vi "Stream to Image Files (Optimized Performance) ajg.vi"() -> ()   [LabVIEW 2020]
doc: "The Stream to Image Files (Optimized Performance) example shows how to save images to PNG files in parallel when using a ring acquisition. Images acquired from a camera are stored in a ring buffer and references to each image are pushed to a queue. Each worker loop removes a reference from the queue and saves the image to disk. When processing is complete, <B>IMAQdx Release Image</B> must be called in order to free space in the ring buffer."
uses:
  <vilib>/vision/driver/IMAQdx.llb/IMAQdx Acquisition Mode.ctl
  <vilib>/vision/Image Controls.llb/IMAQ Image.ctl
  <vilib>/vision/driver/IMAQdx.llb/IMAQdx Buffer Number Mode.ctl
  <vilib>/Utility/High Resolution Relative Seconds.vi
  <vilib>/vision/driver/NI_Vision_Acquisition_Software.lvlib
  <resource>/objmgr/imaqdx.rc
panel:
  in  "Tab Control":enum32{"Main", "Instructions"}(tab)
  in  "Stop":bool
  in  "Camera Name":refnum<k21> caption="IMAQdx Session"
  in  "Number of Images":i32=30
  out "Images Behind":i32
  out "Write Speed":dbl(graph) caption="Image File Write Speed"
  in  "Number of Workers":u8=3 min=1 max=3
  out "Images Acquired Per Second":dbl
  out "Images Saved Per Second":dbl
  in  "Skip Count":u32
  in  "Destination Folder":path
  in  "ms between datasets":dbl
  out "error out 2":errorcluster
  in  "Stopped":bool
  # "Overview: Stream images to disk in parallel. Creates folders within destinatio folder and puts 10,000 files in each folder.\nRequirements: Vision Acquisition Software\nInstructions:\n1. Select the Camera Name\n2. Run the VI\n3. Reduce the Number of Workers to see if the streaming of images can keep up with fewer workers.\n4. Increase the Skip Count if Images Behind is greater than 0.\n5. Use the skip count to skip acquiring some images so the image logging can avoid getting behind.\n6. max workers is 3"
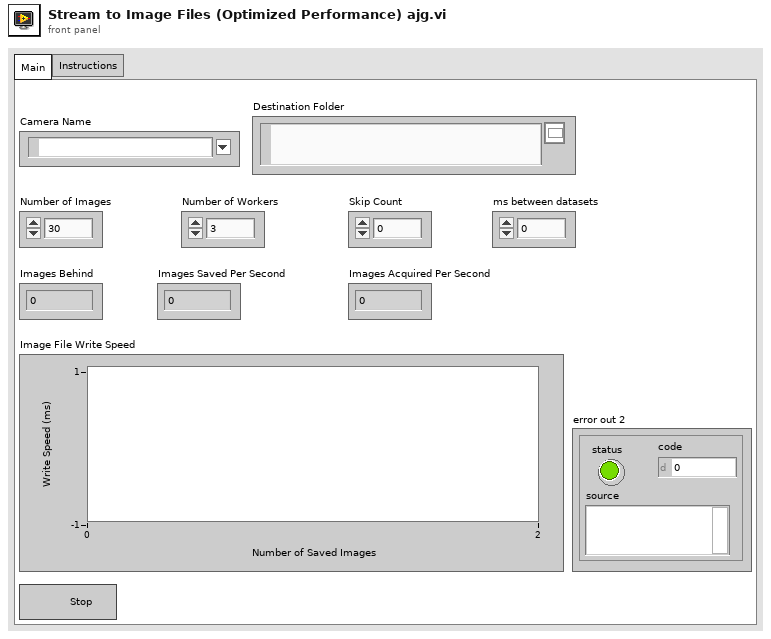
[diagram p1: front panel]
types:
  T1 = typedef "IMAQ Image.ctl" = refnum<image>
  T2 = typedef "NI_Vision_Acquisition_Software.lvlib/IMAQdx Acquisition Mode.ctl" = enum32{"One Shot", "Continuous"}
  T3 = typedef "NI_Vision_Acquisition_Software.lvlib/IMAQdx Buffer Number Mode.ctl" = enum32{"Next", "Last", "Buffer Number", "Every", "Last New"}
  T4 = typedef "IMAQdx.ctl" = refnum<k21>
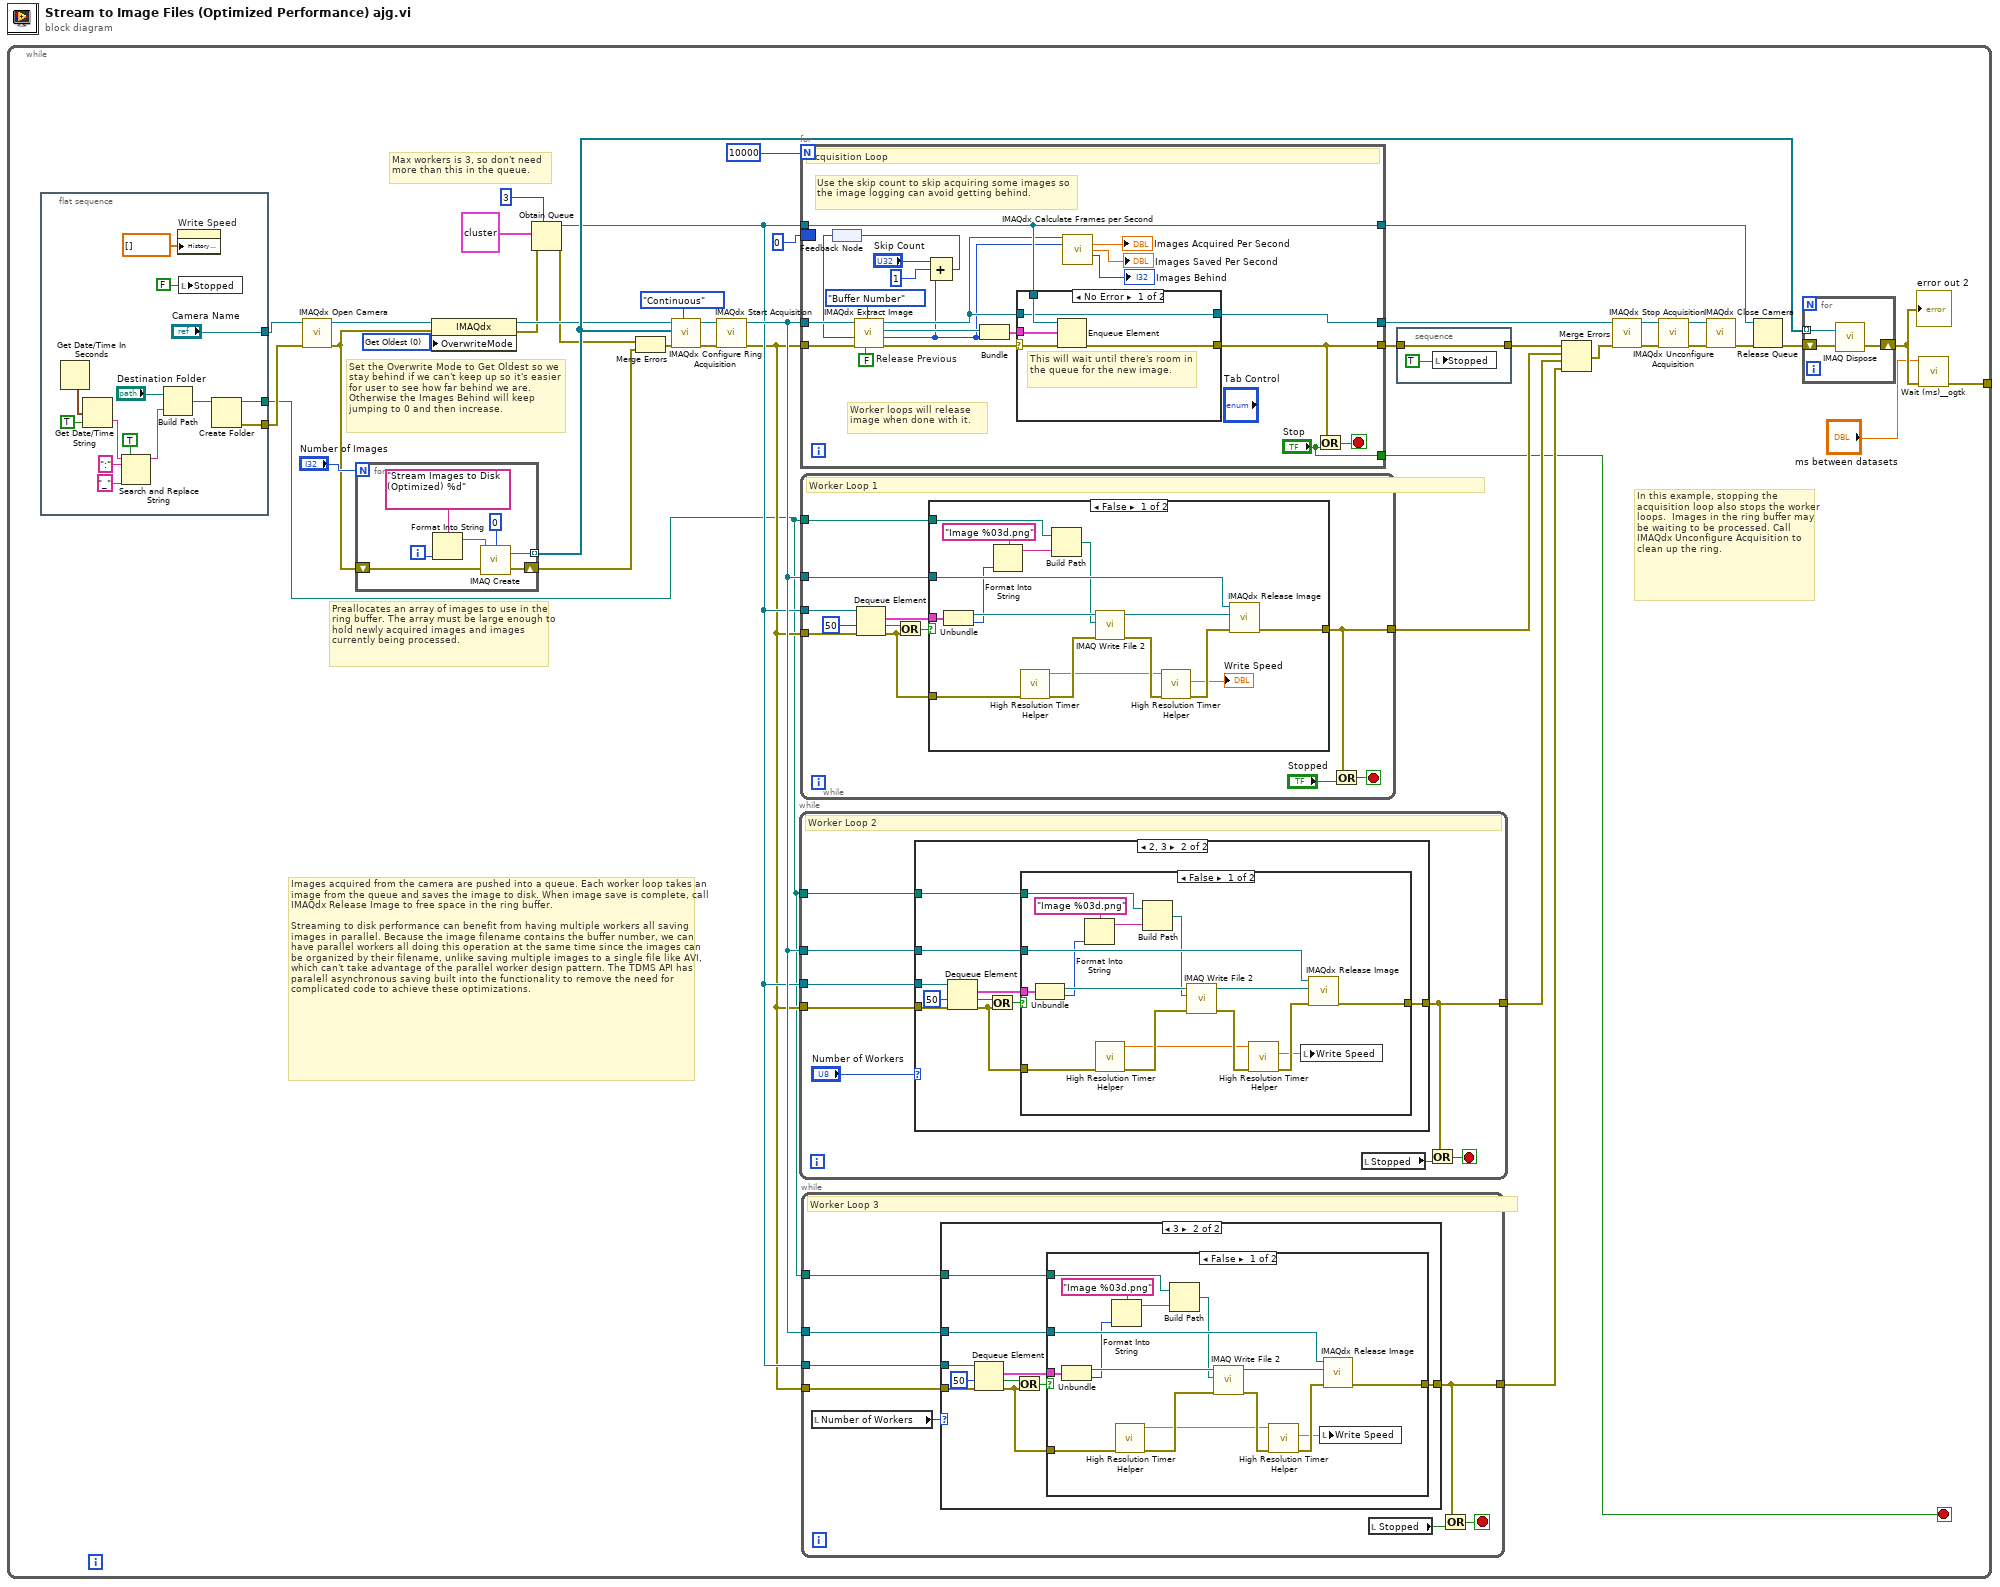
[diagram p0: block diagram]
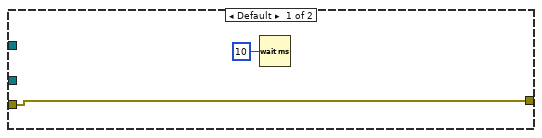
[diagram p3: hidden frame]
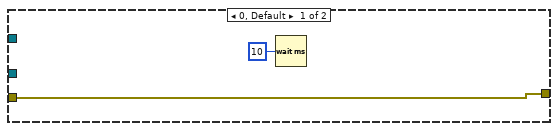
[diagram p5: hidden frame]
diagram:
  n1 = while {
    tunnel: [w3] -> _
    stop <- w10 stop-if-true
    w16 = u32 0 items=["Get Oldest"=0, "Fail"=2, "Get Newest"=3] ("OverwriteMode")
    # "Set the Overwrite Mode to Get Oldest so we stay behind if we can't keep up so it's easier for user to see how far behind we are. Otherwise the Images Behind will keep jumping to 0 and then increase."
    # "Max workers is 3, so don't need more than this in the queue."
    # "In this example, stopping the acquisition loop also stops the worker loops.  Images in the ring buffer may be waiting to be processed. Call IMAQdx Unconfigure Acquisition to clean up the ring."
    # "Images acquired from the camera are pushed into a queue. Each worker loop takes an image from the queue and saves the image to disk. When image save is complete, call IMAQdx Release Image to free space in the ring buffer. \n\nStreaming to disk performance can benefit from having multiple workers all saving images in parallel. Because the image filename contains the buffer number, we can have parallel workers all doing this operation at the same time since the images can be organized by their filename, unlike saving multiple images to a single file like AVI, which can't take advantage of the parallel worker design pattern. The TDMS API has paralell asynchronous saving built into the functionality to remove the need for complicated code to achieve these optimizations."
    # "Preallocates an array of images to use in the ring buffer. The array must be large enough to hold newly acquired images and images currently being processed."
    n2 = flat-sequence {
      tunnel: ["Camera Name"] -> w6
      tunnel: [w42] -> w5
      tunnel: [w41] -> w4
      frame #0 {
        n3 = Get Date/Time In Seconds() -> (seconds since 1Jan1904=w47:timestamp)
        n4 = Get Date/Time String(seconds (now)=w47, want seconds? (F)=TRUE) -> (time string=w48:string)  [unwired: 1 in, 1 out]
        n5 = Search and Replace String(replace all?=TRUE ("replace all? (F)"), input string=w48, search string=":", replace string="_" ("replace string (\"\")")) -> (result string=w51:string)  [unwired: 4 in, 3 out]
        n6 = Build Path(base path="Destination Folder", name or relative path=w51) -> (appended path=w50:path)
        n7 = property on="Write Speed" class="WFChart (strict)"("History Data"=dbl[] []) -> ()  [unwired: 2 in, 2 out]
        n8 = local write "Stopped"(FALSE ("Stop")) -> ()
        n9 = Create Folder(path (use dialog)=w50) -> (created path=w41:path, error out=w42:errorcluster)  [unwired: 2 in, 1 out]
      }
    }
    n10 = call <vilib>:"IMAQdx Open Camera.vi"("error in"=w5, "Session In"=w6) -> ("error out"=w15:errorcluster, "Session Out"=w17:T4)  [unwired: 1 in, 7 out]
    n11 = for {
      N: "Number of Images" -> [_]
      tunnel: [w196] -> w30 mode=indexing
      shift-right: [w195] -> w12
      shift-left: w15 -> [w197]
      i -> [w194]
      n12 = Format Into String(format string="Stream Images to Disk (Optimized) %d" ("Image Name"), w194) -> (resulting string=w193:string)  [unwired: 2 in, 1 out]
      n13 = call "IMAQ Create"("Border Size"=0, "Image Name"=w193, "error in (no error)"=w197) -> ("New Image"=w196:T1, "error out"=w195:errorcluster)  [unwired: 1 in, 1 out]
    }
    n14 = property class="IMAQdx"(reference=w17, error in=w15, "OverwriteMode"=w16) -> (error out=w14:errorcluster)  [unwired: 1 out]
    n15 = Obtain Queue(max queue size (-1, unlimited)=3, element data type=cluster{"Image Out":T1, "Buffer Number Out":u32} {"Image Out"=refnum, "Buffer Number Out"=0}, error in (no error)=w14) -> (queue out=w21:refnum<queue>, error out=w13:errorcluster)  [unwired: 2 in, 1 out]
    n16 = Merge Errors(w13, w12) -> (w33:errorcluster)
    n17 = call <vilib>:"IMAQdx Configure Ring Acquisition.vi"("Mode"=IMAQdx_Acquisition_Mode."Continuous" ("Continuous?"), "error in"=w33, "Images"=w30, "Session In"=w17) -> ("error out"=w9:errorcluster, "Session Out"=w36:T4)  [unwired: 5 in, 1 out]
    n18 = call <vilib>:"IMAQdx Start Acquisition.vi"("error in"=w9, "Session In"=w36) -> ("error out"=w20:errorcluster, "Session Out"=w22:T4)  [unwired: 8 out]
    n19 = while {
      tunnel: w21 -> [w124]
      tunnel: w22 -> [w126]
      tunnel: w20 -> [w123]
      tunnel: w4 -> [w125]
      tunnel: [w122] -> w23
      stop <- w127 stop-if-true
      # "Worker Loop 2"
      n20 = case shown="2, 3" "Number of Workers" {
        tunnel: w126 -> [_ w134]
        tunnel: w125 -> [_ w133]
        tunnel: w124 -> [_ w132]
        tunnel: w123 -> [w129 w131]
        tunnel: [w129 w130] -> w122
        frame 0, Default {
          n21 = Wait (ms)(milliseconds to wait=u32 10) -> ()  [unwired: 1 out]
        }
        frame 2, 3 {
          n22 = Dequeue Element(queue=w132, timeout in ms (-1)=50 ("timeout in ms"), error in (no error)=w131) -> (element=w136:cluster{"Image Out":T1, "Buffer Number Out":u32}, timed out?=w138:bool, error out=w139:errorcluster)  [unwired: 1 out]
          n23 = Or(x=w138, y=w139) -> (x .or. y?=w137:bool)
          n24 = case shown="False" w137 {
            tunnel: w139 -> [w145 w156]
            tunnel: w136 -> [w155 _]
            tunnel: [w154 w156] -> w130
            tunnel: w134 -> [w153 _]
            tunnel: w133 -> [w150 _]
            frame False {
              n25 = Unbundle(w155) -> ("Image Out"=w152:T1, "Buffer Number Out"=w147:u32)
              n26 = Format Into String(format string="Image %03d.png", w147) -> (resulting string=w149:string)  [unwired: 2 in, 1 out]
              n27 = call "High Resolution Timer Helper.vi"("error in (no error)"=w145) -> ("error out"=w144:errorcluster, "Current Time"=w141:dbl)  [unwired: 8 in, 1 out]
              n28 = Build Path(base path=w150, name or relative path=w149) -> (appended path=w146:path)
              n29 = call-poly "IMAQ Write File 2"("error in (no error)"=w144, "File Path"=w146, "Image"=w152) -> ("error out"=w143:errorcluster, "Image Out (duplicate)"=w151:T1)  [unwired: 7 in]
              n30 = call "High Resolution Timer Helper.vi"("error in (no error)"=w143, "Previous Time"=w141) -> ("error out"=w142:errorcluster, "Time Difference (ms)"=w140:dbl)  [unwired: 7 in, 1 out]
              n31 = local write "Write Speed"(w140) -> ()
              n32 = call <vilib>:"IMAQdx Release Image.vi"("error in"=w142, "Image"=w151, "Session In"=w153) -> ("error out"=w154:errorcluster)  [unwired: 7 in, 1 out]
            }
            frame True {
              # "Empty queue or error.\nNothing to process."
            }
          }
        }
      }
      n33 = local read "Stopped"() -> (w120:bool)
      n34 = Or(x=w122, y=w120) -> (x .or. y?=w127:bool)
    }
    n35 = for {
      N: 10000 ("Max Files") -> [_]
      tunnel: w20 -> [w75]
      tunnel: w22 -> [w72]
      tunnel: w21 -> [w68]
      tunnel: [w67] -> w29
      tunnel: [w66] -> w26
      tunnel: [w68] -> w31
      tunnel: ["Stop"] -> w10
      border: u32 0 -> [_]
      stop <- w56 stop-if-true
      w73 = FALSE  # Release Previous
      # "Use the skip count to skip acquiring some images so the image logging can avoid getting behind."
      # "Worker loops will release image when done with it."
      # "Acquisition Loop"
      n36 = feedback #1() -> (w64:u32)
      n37 = call <vilib>:"IMAQdx Extract Image.vi"("Release Previous (true)"=w73, "Buffer Number Mode (Next)"=IMAQdx_Buffer_Number_Mode."Buffer Number" ("Buffer Number Mode"), "error in"=w75, "Buffer Number In"=w64, "Session In"=w72) -> ("error out"=w71:errorcluster, "Buffer Number Out"=w57:u32, "Image Out"=w70:T1, "Session Out"=w58:T4)  [unwired: 3 in]
      n38 = Compound Arithmetic op=ADD("Skip Count", u32 1 ("value"), w57) -> (w65:u32)
      n39 = feedback-in #1(w65) -> ()
      n40 = Bundle("Image Out"=w70, "Buffer Number Out"=w57) -> (w69:cluster{"Image Out":T1, "Buffer Number Out":u32})  [unwired: 1 in]
      n41 = case shown="No Error" w71 {
        selector: w71 -> [w80 w81]
        tunnel: [w76 w82] -> w67
        tunnel: w58 -> [w76 w82]
        tunnel: w69 -> [w79 _]
        tunnel: w68 -> [w78 _]
        tunnel: [w77 w81] -> w66
        frame No Error {
          # "This will wait until there's room in the queue for the new image."
          n42 = Enqueue Element(queue=w78, element=w79, error in (no error)=w80) -> (error out=w77:errorcluster)  [unwired: 1 in, 2 out]
        }
        frame Error {
        }
      }
      n43 = call <vilib>:"IMAQdx Calculate Frames per Second.vi"("Session In"=w58, "Buffer Number"=w57) -> ("Acquired Frames per Second"=→"Images Acquired Per Second":dbl, "Processed Frames per Second"=→"Images Saved Per Second":dbl, "Images Behind"=→"Images Behind":i32)  [unwired: 7 in, 4 out]
      n44 = Or(x=w66, y="Stop") -> (x .or. y?=w56:bool)
    }
    n45 = while {
      tunnel: w21 -> [w165]
      tunnel: w22 -> [w167]
      tunnel: w20 -> [w164]
      tunnel: w4 -> [w166]
      tunnel: [w163] -> w24
      stop <- w173 stop-if-true
      # "Worker Loop 1"
      n46 = Dequeue Element(queue=w165, timeout in ms (-1)=50 ("timeout in ms"), error in (no error)=w164) -> (element=w169:cluster{"Image Out":T1, "Buffer Number Out":u32}, timed out?=w171:bool, error out=w172:errorcluster)  [unwired: 1 out]
      n47 = Or(x=w171, y=w172) -> (x .or. y?=w170:bool)
      n48 = case shown="False" w170 {
        tunnel: w172 -> [w179 w190]
        tunnel: w169 -> [w189 _]
        tunnel: [w188 w190] -> w163
        tunnel: w167 -> [w187 _]
        tunnel: w166 -> [w184 _]
        frame False {
          n49 = Unbundle(w189) -> ("Image Out"=w186:T1, "Buffer Number Out"=w181:u32)
          n50 = Format Into String(format string="Image %03d.png", w181) -> (resulting string=w183:string)  [unwired: 2 in, 1 out]
          n51 = call "High Resolution Timer Helper.vi"("error in (no error)"=w179) -> ("error out"=w178:errorcluster, "Current Time"=w176:dbl)  [unwired: 8 in, 1 out]
          n52 = Build Path(base path=w184, name or relative path=w183) -> (appended path=w180:path)
          n53 = call-poly "IMAQ Write File 2"("error in (no error)"=w178, "File Path"=w180, "Image"=w186) -> ("error out"=w177:errorcluster, "Image Out (duplicate)"=w185:T1)  [unwired: 7 in]
          n54 = call "High Resolution Timer Helper.vi"("error in (no error)"=w177, "Previous Time"=w176) -> ("error out"=w175:errorcluster, "Time Difference (ms)"=→"Write Speed":dbl)  [unwired: 7 in, 1 out]
          n55 = call <vilib>:"IMAQdx Release Image.vi"("error in"=w175, "Image"=w185, "Session In"=w187) -> ("error out"=w188:errorcluster)  [unwired: 7 in, 1 out]
        }
        frame True {
          # "Empty queue or error.\nNothing to process."
        }
      }
      n56 = Or(x=w163, y="Stopped") -> (x .or. y?=w173:bool)
    }
    n57 = while {
      tunnel: w21 -> [w87]
      tunnel: w22 -> [w89]
      tunnel: w20 -> [w86]
      tunnel: w4 -> [w88]
      tunnel: [w85] -> w19
      stop <- w90 stop-if-true
      # "Worker Loop 3"
      n58 = local read "Number of Workers"() -> (w84:u8)
      n59 = case shown="3" w84 {
        tunnel: w89 -> [_ w97]
        tunnel: w88 -> [_ w96]
        tunnel: w87 -> [_ w95]
        tunnel: w86 -> [w92 w94]
        tunnel: [w92 w93] -> w85
        frame Default {
          n60 = Wait (ms)(milliseconds to wait=u32 10) -> ()  [unwired: 1 out]
        }
        frame 3 {
          n61 = Dequeue Element(queue=w95, timeout in ms (-1)=50 ("timeout in ms"), error in (no error)=w94) -> (element=w99:cluster{"Image Out":T1, "Buffer Number Out":u32}, timed out?=w101:bool, error out=w102:errorcluster)  [unwired: 1 out]
          n62 = Or(x=w101, y=w102) -> (x .or. y?=w100:bool)
          n63 = case shown="False" w100 {
            tunnel: w102 -> [w108 w119]
            tunnel: w99 -> [w118 _]
            tunnel: [w117 w119] -> w93
            tunnel: w97 -> [w116 _]
            tunnel: w96 -> [w113 _]
            frame False {
              n64 = Unbundle(w118) -> ("Image Out"=w115:T1, "Buffer Number Out"=w110:u32)
              n65 = Format Into String(format string="Image %03d.png", w110) -> (resulting string=w112:string)  [unwired: 2 in, 1 out]
              n66 = call "High Resolution Timer Helper.vi"("error in (no error)"=w108) -> ("error out"=w107:errorcluster, "Current Time"=w105:dbl)  [unwired: 8 in, 1 out]
              n67 = Build Path(base path=w113, name or relative path=w112) -> (appended path=w109:path)
              n68 = call-poly "IMAQ Write File 2"("error in (no error)"=w107, "File Path"=w109, "Image"=w115) -> ("error out"=w106:errorcluster, "Image Out (duplicate)"=w114:T1)  [unwired: 7 in]
              n69 = call "High Resolution Timer Helper.vi"("error in (no error)"=w106, "Previous Time"=w105) -> ("error out"=w104:errorcluster, "Time Difference (ms)"=w103:dbl)  [unwired: 7 in, 1 out]
              n70 = local write "Write Speed"(w103) -> ()
              n71 = call <vilib>:"IMAQdx Release Image.vi"("error in"=w104, "Image"=w114, "Session In"=w116) -> ("error out"=w117:errorcluster)  [unwired: 7 in, 1 out]
            }
            frame True {
              # "Empty queue or error.\nNothing to process."
            }
          }
        }
      }
      n72 = local read "Stopped"() -> (w83:bool)
      n73 = Or(x=w85, y=w83) -> (x .or. y?=w90:bool)
    }
    n74 = stacked-sequence {
      tunnel: [w158] -> w25
      tunnel: w26 -> [w158]
      frame #0 {
        n75 = local write "Stopped"(TRUE ("Stop")) -> ()
      }
    }
    n76 = Merge Errors(w25, w24, w23, w19) -> (w1:errorcluster)
    n77 = call <vilib>:"IMAQdx Stop Acquisition.vi"("error in"=w1, "Session In"=w29) -> ("error out"=w37:errorcluster, "Session Out"=w38:T4)  [unwired: 8 out]
    n78 = call <vilib>:"IMAQdx Unconfigure Acquisition.vi"("error in"=w37, "Session In"=w38) -> ("error out"=w40:errorcluster, "Session Out"=w39:T4)  [unwired: 8 out]
    n79 = call <vilib>:"IMAQdx Close Camera.vi"("error in"=w40, "Session In"=w39) -> ("error out"=w28:errorcluster)  [unwired: 9 out]
    n80 = Release Queue(queue=w31, error in (no error)=w28) -> (error out=w27:errorcluster)  [unwired: 1 in, 2 out]
    n81 = for {
      shift-right: [w160] -> w8
      shift-left: w27 -> [w161]
      tunnel: w30 -> [w159] mode=indexing
      n82 = call "IMAQ Dispose"("Image"=w159, "error in (no error)"=w161) -> ("error out"=w160:errorcluster)  [unwired: 4 in]
    }
    "error out 2" <- w8
    n83 = call <userlib>:"Wait (ms)__ogtk.vi"("error in (no error)"=w8, "milliseconds to wait"="ms between datasets") -> ("error out"=w3:errorcluster)  [unwired: 8 in, 1 out]
  }
